vi "Read Timeout Message.vi"(8 "error in (no error)":errorcluster, 11 "IEventHandler in":refnum<class "IEventHandler.lvclass">) -> (0 "error out":errorcluster, 2 "Timeout Message":refnum<class "Message.lvclass">, 3 "IEventHandler out":refnum<class "IEventHandler.lvclass">)   [LabVIEW 2017, in "ActorEvents.lvlib" / "IEventHandler.lvclass"]
uses:
  <vilib>/gpm_packages/@cs/mva-viewable/Source/ActorEvents/IEventHandler/IEventHandler.lvclass
  <vilib>/ActorFramework/Message/Message.lvclass
  <vilib>/gpm_packages/@cs/mva-viewable/Source/ActorEvents/IEventHandler/IEventHandler.lvclass/IEventHandler.ctl
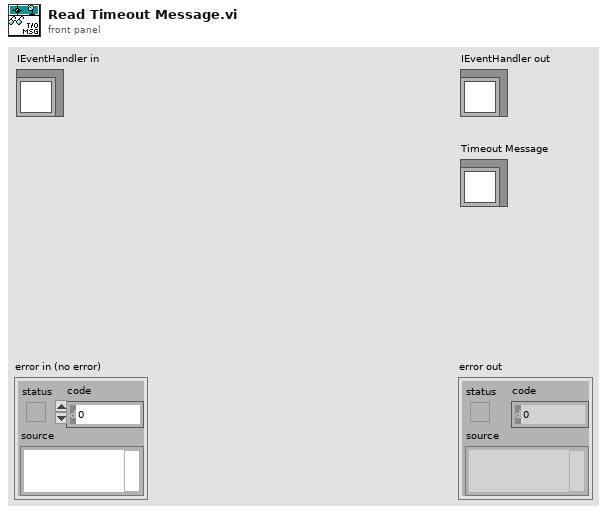
[diagram p1: front panel]
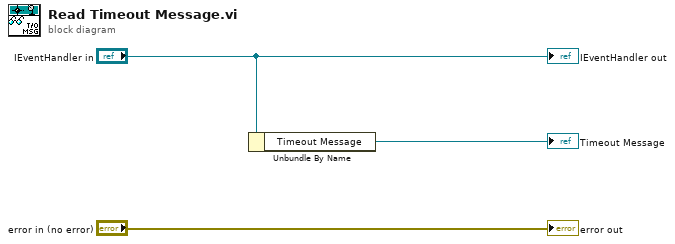
[diagram p0: block diagram]
diagram:
  n1 = Unbundle By Name("IEventHandler in") -> ("Timeout Message"=→"Timeout Message":refnum<class "Message.lvclass">)
  "error out" <- "error in (no error)"
  "IEventHandler out" <- "IEventHandler in"
